vi "Write To CSV File.vi"(8 "Values":dbl[][](array[numeric]), 9 "Names":string[](array[string]), 10 "Output Directory":path=path "C:/Users/Josh/Desktop/code/CVB/Config/generated_data", 11 "Create New File":bool) -> (3 "Output Filename":path)   [LabVIEW 2021]
uses:
  <vilib>/Utility/file.llb/Write Delimited Spreadsheet (string).vi
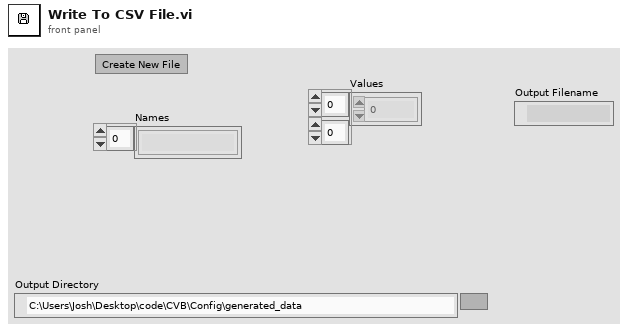
[diagram p1: front panel]
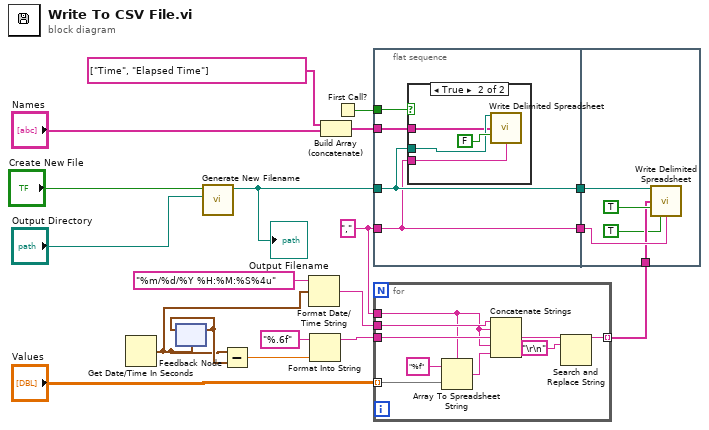
[diagram p0: block diagram]
diagram:
  w11 = "," ("delimiter (\\t)")
  n1 = Get Date/Time In Seconds() -> (seconds since 1Jan1904=w6:timestamp)
  n2 = feedback #1(w6) -> (w7:timestamp)
  n3 = feedback-in #1(w7) -> ()
  n4 = call "Generate New Filename.vi"("Output Directory"="Output Directory", "Create New File"="Create New File") -> ("Output Filename"=w4:path)  [unwired: 9 in]
  "Output Filename" <- w4
  n5 = Subtract(x=w6, y=w7) -> (x-y=w8:dbl)
  n6 = Format Date/Time String(time format string (%c)="%m/%d/%Y %H:%M:%S%4u", seconds (now)=w6) -> (date/time string=w10:string)  [unwired: 1 in]
  n7 = Format Into String(format string="%.6f", w8) -> (resulting string=w12:string)  [unwired: 2 in, 1 out]
  n8 = Build Array (concatenate)(string[] ["Time", "Elapsed Time"] ("array"), "Names") -> (w15:string[])
  n9 = First Call?() -> (First Call?: T/F=w3:bool)
  n10 = flat-sequence {
    tunnel: w15 -> [w23]
    tunnel: w3 -> [w22]
    tunnel: w4 -> [w21]
    tunnel: [w21] -> w19
    tunnel: w11 -> [w20]
    tunnel: [w20] -> w18
    tunnel: w19 -> [w31]
    tunnel: w18 -> [w30]
    tunnel: w13 -> [w29]
    frame #0 {
      n11 = case shown="True" w22 {
        tunnel: w23 -> [_ w24]
        tunnel: w21 -> [_ w26]
        tunnel: w20 -> [_ w25]
        frame False {
        }
        frame True {
          n12 = call-poly <vilib>:"Write Delimited Spreadsheet.vi"("file path (dialog if empty)"=w26, "1D data"=w24, "append to file? (new file:F)"=FALSE, "delimiter (\\t)"=w25) -> ()  [unwired: 10 in, 2 out]
        }
      }
    }
    frame #1 {
      n13 = call-poly <vilib>:"Write Delimited Spreadsheet.vi"("file path (dialog if empty)"=w31, "1D data"=w29, "append to file? (new file:F)"=TRUE, "transpose? (no:F)"=TRUE, "delimiter (\\t)"=w30) -> ()  [unwired: 9 in, 2 out]
    }
  }
  n14 = for {
    tunnel: w10 -> [w37]
    tunnel: w11 -> [w33]
    tunnel: w12 -> [w34]
    tunnel: [w36] -> w13 mode=indexing
    tunnel: "Values" -> [w35] mode=indexing
    n15 = Array To Spreadsheet String(delimiter (Tab)=w33, array=w35, 3:"%f" ("format string")) -> (spreadsheet string=w40:string)
    n16 = Concatenate Strings(w37, w33, w34, w33, w40) -> (w39:string)
    n17 = Search and Replace String(input string=w39, search string="\r\n") -> (result string=w36:string)  [unwired: 6 in, 3 out]
  }
